vi "Create Queues.vi"(8 "error in (no error)":errorcluster) -> (0 "error out":errorcluster)   [LabVIEW 2017, in "Akwizycja.lvlib"]
uses:
  Akwizycja.lvlib
panel:
  in  "TLS Cluster":T1
  in  "Fuel Flows":dbl[][](array[numeric])
  in  "Avg fuel":T2
  in  "output cluster":T2
  in  "Array in":dbl[][](array[numeric])
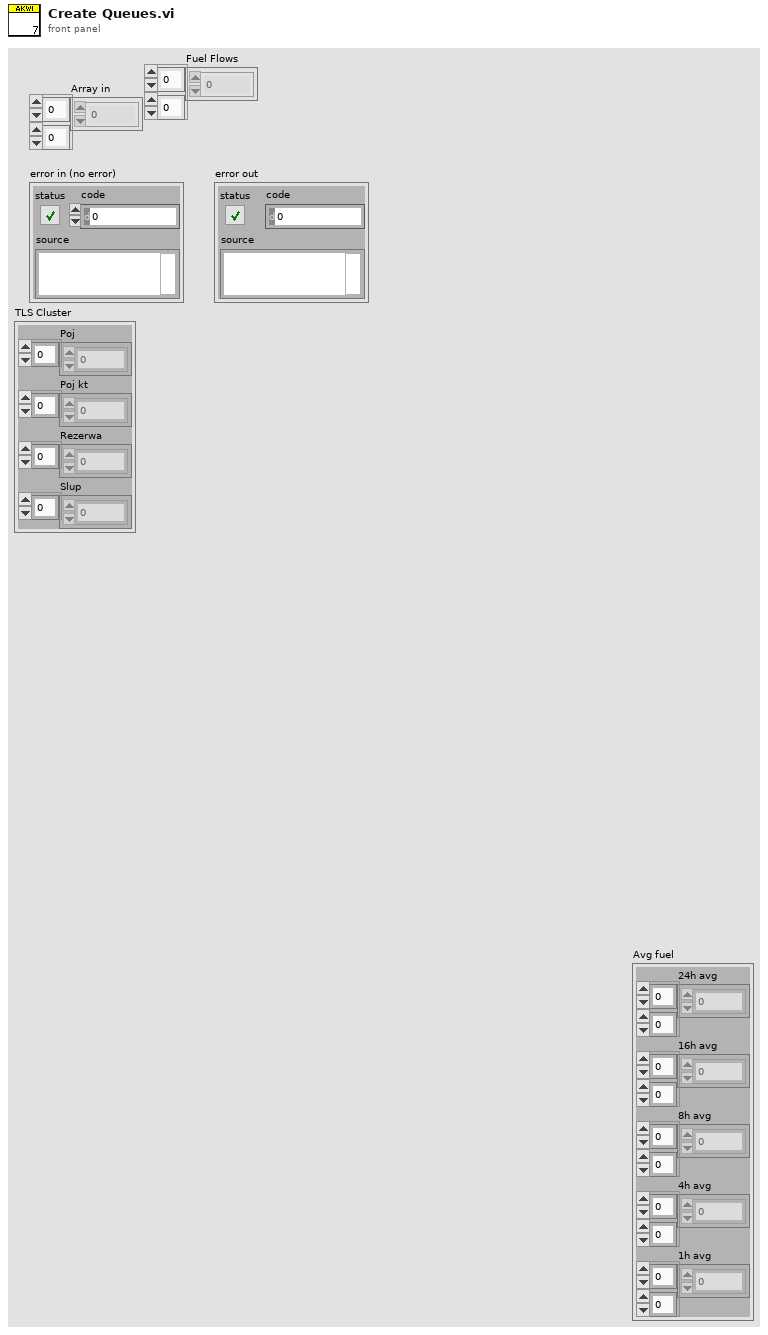
[diagram p1: front panel]
types:
  T1 = cluster{"Poj":sgl[], "Poj kt":sgl[], "Rezerwa":sgl[], "Slup":sgl[]}
  T2 = cluster{"24h avg":dbl[][], "16h avg":dbl[][], "8h avg":dbl[][], "4h avg":dbl[][], "1h avg":dbl[][]}
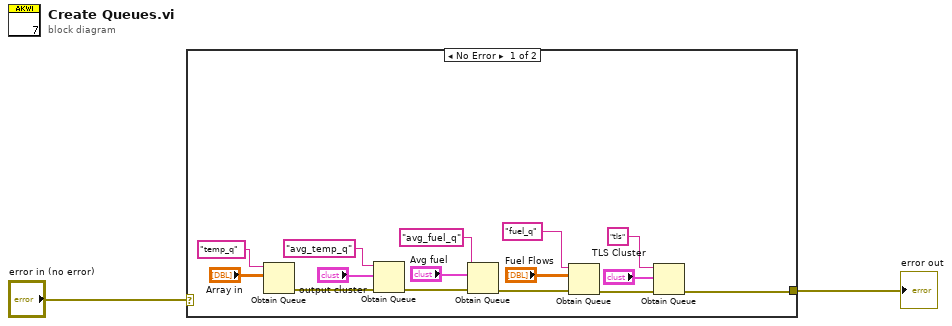
[diagram p0: block diagram]
diagram:
  n1 = case shown="No Error" "error in (no error)" {
    selector: "error in (no error)" -> [_ w18]
    tunnel: [w5 w18] -> w2
    frame No Error {
      n2 = Obtain Queue(name (unnamed)="temp_q", element data type="Array in") -> (error out=w13:errorcluster)  [unwired: 3 in, 2 out]
      n3 = Obtain Queue(name (unnamed)="avg_temp_q", element data type="output cluster", error in (no error)=w13) -> (error out=w10:errorcluster)  [unwired: 2 in, 2 out]
      n4 = Obtain Queue(name (unnamed)="avg_fuel_q", element data type="Avg fuel", error in (no error)=w10) -> (error out=w8:errorcluster)  [unwired: 2 in, 2 out]
      n5 = Obtain Queue(name (unnamed)="fuel_q", element data type="Fuel Flows", error in (no error)=w8) -> (error out=w6:errorcluster)  [unwired: 2 in, 2 out]
      n6 = Obtain Queue(name (unnamed)="tls", element data type="TLS Cluster", error in (no error)=w6) -> (error out=w5:errorcluster)  [unwired: 2 in, 2 out]
    }
    frame Error {
    }
  }
  "error out" <- w2
